vi "Read Bus Controller and Acyclic Frames.vi"(8 "error in":errorcluster, 11 "port in":T1 format="%.0x") -> (0 "error out":errorcluster, 1 "bus controller name":string, 2 "bus controller found":bool=TRUE, 3 "port out":T1 format="%.0x", 4 "acyclic frame names":string[](array[string]))   [LabVIEW 2020, in "Ballard MIL-STD-1553 Scripting.lvlib"]
uses:
  <vilib>/NI VeriStand/Custom Device API/Custom Device Item Ref.ctl
  Constants.vi
  <vilib>/NI VeriStand/Custom Device Tools/Custom Device Utility Library/NI VeriStand - Search for All Items by GUID.vi
  <vilib>/NI VeriStand/Custom Device API/Get Item Property (String).vi
  Ballard MIL-STD-1553 Scripting.lvlib
  <vilib>/NI VeriStand/Custom Device Tools/Custom Device Utility Library/Custom Device Utility Library.lvlib
  <vilib>/NI VeriStand/Custom Device API/Custom Device API.lvlib
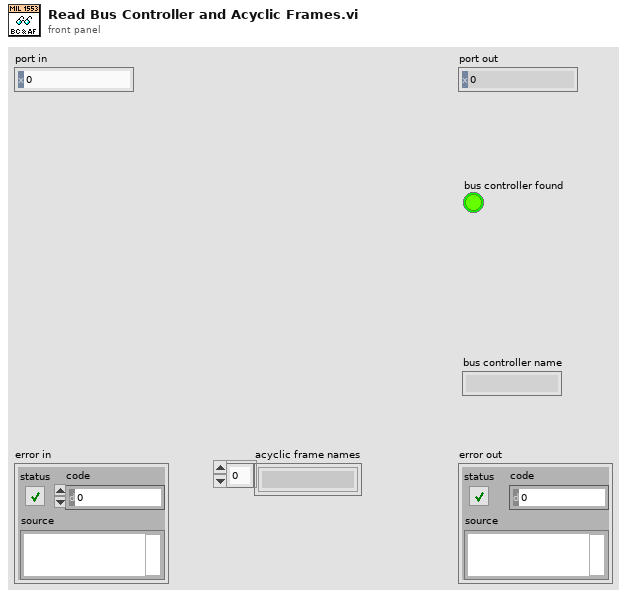
[diagram p1: front panel]
types:
  T1 = typedef "Custom Device API.lvlib/Custom Device Item Ref.ctl" = u64
  T2 = typedef "Custom Device API.lvlib/Custom Device Item Info.ctl" = cluster{"Name":string, "Is Channel":bool, "GUID":string, "Is Waveform":bool}
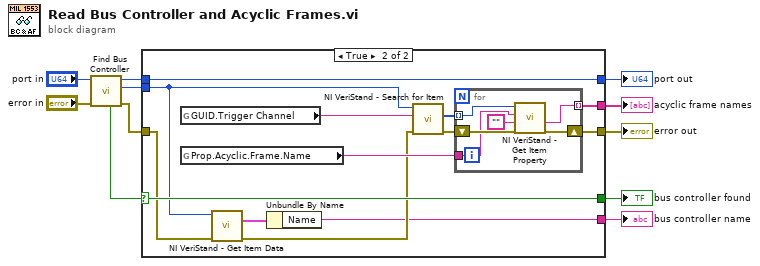
[diagram p0: block diagram]
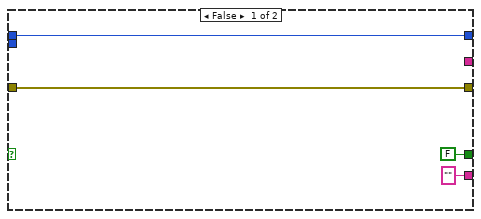
[diagram p2: hidden frame]
diagram:
  n1 = call "Find Bus Controller.vi"("error in"="error in", "port in"="port in") -> ("error out"=w8:errorcluster, "bus controller"=w9:T1, "port out"=w6:T1, "found?"=w7:bool)  [unwired: 6 in]
  n2 = case shown="True" w7 {
    selector: w7 -> [_ w21]
    tunnel: w6 -> [w15 w28]
    tunnel: w8 -> [w14 w19]
    tunnel: [w15 w28] -> w5
    tunnel: [w14 w23] -> w10
    tunnel: w9 -> [_ w20]
    tunnel: [_ w22] -> w11
    tunnel: [FALSE w21] -> w4
    tunnel: ["" ("Name") w16] -> w3
    frame False {
    }
    frame True {
      n3 = global read "Constants.vi" "GUID.Trigger Channel"() -> (w27:string)
      n4 = global read "Constants.vi" "Prop.Acyclic.Frame.Name"() -> (w24:string)
      n5 = call <vilib>:"NI VeriStand - Get Item Data.vi"("error in (no error)"=w19, "Item Ref in"=w20) -> ("error out"=w18:errorcluster, "Item Info"=w17:T2)  [unwired: 6 in, 2 out]
      n6 = Unbundle By Name(w17) -> ("Name"=w16:string)
      n7 = call-poly <vilib>:"NI VeriStand - Search for Item.vi"("error in"=w18, "Item GUID"=w27, "Section Ref in"=w20) -> ("error out"=w25:errorcluster, "Item Refs"=w26:T1[])  [unwired: 5 in, 2 out]
      n8 = for {
        tunnel: w26 -> [w33] mode=indexing
        shift-right: [w34] -> w23
        shift-left: w25 -> [w32]
        tunnel: w24 -> [w31]
        tunnel: [w29] -> w22 mode=indexing
        n9 = call-poly <vilib>:"NI VeriStand - Get Item Property.vi"("error in (no error)"=w32, "Default Value"="", "Property Name"=w31, "Item Ref in"=w33) -> ("error out"=w34:errorcluster, "Value"=w29:string)  [unwired: 4 in, 2 out]
      }
    }
  }
  "acyclic frame names" <- w11
  "error out" <- w10
  "port out" <- w5
  "bus controller name" <- w3
  "bus controller found" <- w4
